vi "PathPlanner_EventMarker_GetCommand.vi"(11 "in EventMarker":T3) -> (3 "Command":T1)   [LabVIEW 2019, in "PathPlanner24.lvlib"]
doc: "Get the command associated with this marker\n\nInputs:\n - EventMarker - cluster - Data cluster\n\nOutputs:\n - Command - cluster - command for this marker"
uses:
  PathPlanner24.lvlib
  TypeDef/PathPlannerEventMarker.ctl
  TypeDef/PathPlannerCommandUtil.ctl
  ENum/PathPlanner_CommandUtilType_ENUM.ctl
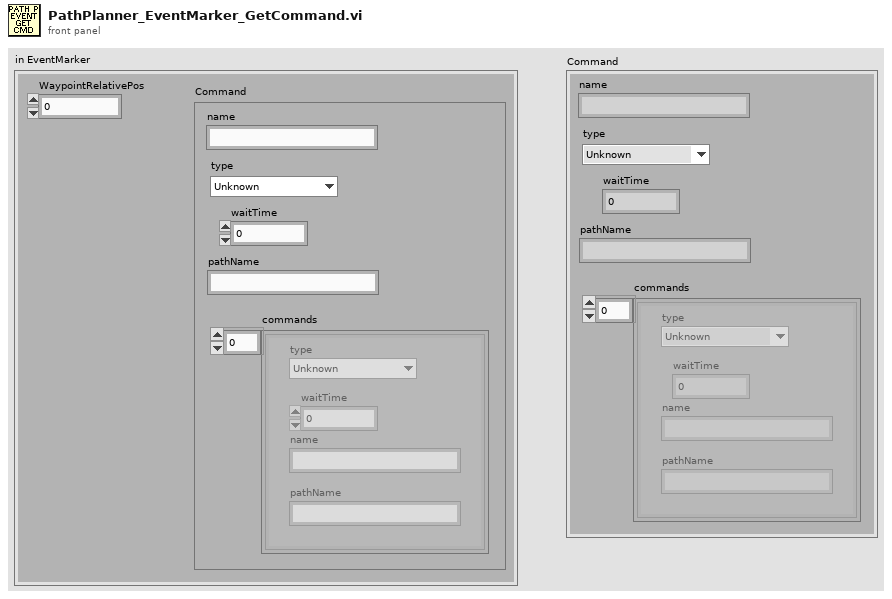
[diagram p1: front panel]
types:
  T1 = typedef "PathPlanner24.lvlib/PathPlannerCommandUtil.ctl" = cluster{"waitTime":dbl, "name":string, "pathName":string, "commands":cluster{"type":T2, "waitTime":dbl, "name":string, "pathName":string}[], "type":T2}
  T2 = typedef "PathPlanner24.lvlib/PathPlanner_CommandUtilType_ENUM.ctl" = enum16{"Unknown", "Wait", "Named", "Path", "Sequential", "Parallel", "Race", "Deadline"}
  T3 = typedef "PathPlanner24.lvlib/PathPlannerEventMarker.ctl" = cluster{"WaypointRelativePos":dbl, "Command":T1}
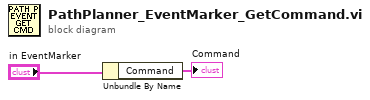
[diagram p0: block diagram]
diagram:
  n1 = Unbundle By Name("in EventMarker") -> ("Command"=→"Command":T1)
